vi "Main.vi"() -> ()   [LabVIEW 2015, in "ISA010_module.lvlib"]
doc: "This template is based from the Queued Message Handler design pattern and the Queued Message Handler Project Template that ships with LabVIEW 2014.\n\nThe main difference is that the Queue is private to this module and communication between modules is done via Broadcast and Requests events.\n\nRequests events are wrapped via public API methods and are handled in the Event handler loop in this VI.\nAny module can register for Broadcast events sent by this module.\n\nThe Event Handling Loop generates messages based on user interface actions.\n\nThe Message Handling Loop processes messages generated by the Event Handling Loop, or by other messages. The messages are string values, so new messages can be added easily to the Message Cases case structure in the Message Handling Loop. Each message cluster can also provide an optional value for Message Data, which is a variant that can be converted to whatever message-specific data is required.\n_____\nBased on Delacor QMH Project Template 3.1.0.34."
uses:
  ISA010_module.lvlib
  <vilib>/Delacor/Delacor QMH/Libraries/Cloneable Module Admin_class/Delacor_lib_QMH_Cloneable Module Admin.lvclass
  Module Data--cluster.ctl
  ISA010/ISA010.lvclass
  libraries/ModBUS.lvlibp/ASCII/ASCII.lvclass
  <vilib>/Delacor/Delacor QMH/Libraries/Cloneable Module Admin_class/Delacor_lib_QMH_Cloneable Module Admin.lvclass/Delacor_lib_QMH_Cloneable Module Admin.ctl
  Stop Argument--cluster.ctl
  <vilib>/Delacor/Delacor QMH/Libraries/Module Admin_class/Delacor_lib_QMH_Module Admin.lvclass/Delacor_lib_QMH_Module Admin.ctl
  getISA010State Argument--cluster.ctl
  setPWM Argument--cluster.ctl
  SetServiceMode Argument--cluster.ctl
  setDKG Argument--cluster.ctl
  setKASAWAR Argument--cluster.ctl
  Config Argument--cluster.ctl
  <vilib>/Utility/miscctls.llb/LVPointTypeDef.ctl
  <vilib>/Delacor/Delacor QMH/Libraries/Cloneable Module Admin_class/Delacor_lib_QMH_Get Module ID.vi
  <vilib>/Delacor/Delacor QMH/Libraries/Module Admin_class/Delacor_lib_QMH_Get External Launch.vi
  <vilib>/Delacor/Delacor QMH/Libraries/Message Queue_class/Delacor_lib_QMH_Enqueue Message (Single).vi
  <vilib>/Utility/error.llb/Error Cluster From Error Code.vi
  <vilib>/ErrorRing/Error Ring.xnode
  <vilib>/Delacor/Delacor QMH/Libraries/Message Queue_class/Delacor_lib_QMH_Message Queue.lvclass
  Clone Registration/Clone Registration.lvlib
  libraries/Serializer.lvlibp
  libraries/MQTT.lvlibp
panel:
  in  "Simulate MHL Error":bool
  in  "Simulate EHL Error":bool
  out "error out":errorcluster
  in  "Module Admin":refnum<class "Delacor_lib_QMH_Cloneable Module Admin.lvclass">
  out "Status":string
  # "Other QMH Modules communicate with this Module via its Public API (wrappers for its Request Events).\n\nThis Module communicates with other Modules via its Broadcast Events.\nAny module that wants to get these messages, just registers for this module's Broadcast events."
  # "This template is for the Delacor Modified Queued Message Handler design pattern.\n\nSee the block diagram for more information on how to use this template."
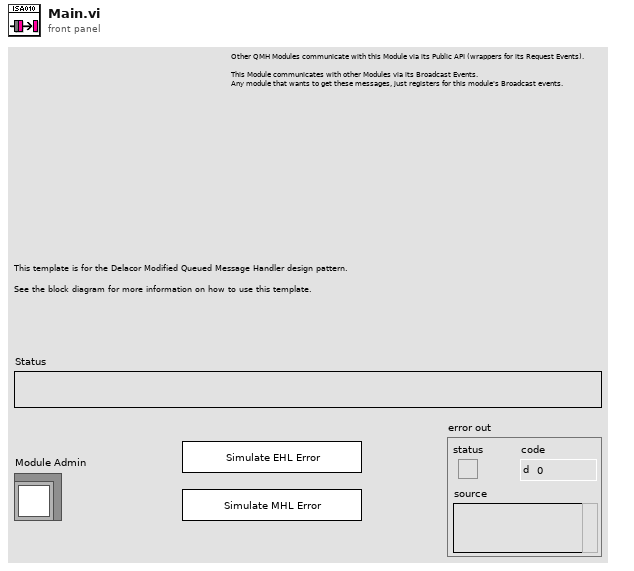
[diagram p1: front panel]
types:
  T1 = typedef "ISA010_module.lvlib/Request Events--cluster.ctl" = cluster{"Stop Module":refnum<user-event>, "Show Panel":refnum<user-event>, "Hide Panel":refnum<user-event>, "Show Diagram":refnum<user-event>, "Get Module Execution Status":refnum<user-event>, "getISA010State":refnum<user-event>, "setPWM":refnum<user-event>, "SetServiceMode":refnum<user-event>, "setDKG":refnum<user-event>, "setKASAWAR":refnum<user-event>, "Config":refnum<user-event>}
  T2 = typedef "Serializer.lvlibp/Broadcast Events--cluster.ctl" = cluster{"Module Did Init":refnum<user-event>, "Status Updated":refnum<user-event>, "Error Reported":refnum<user-event>, "Module Did Stop":refnum<user-event>, "Update Module Execution Status":refnum<user-event>, "Received":refnum<user-event>}
  T3 = typedef "MQTT.lvlibp/Broadcast Events--cluster.ctl" = cluster{"Module Did Init":refnum<user-event>, "Status Updated":refnum<user-event>, "Error Reported":refnum<user-event>, "Module Did Stop":refnum<user-event>, "Update Module Execution Status":refnum<user-event>, "Message":refnum<user-event>}
  T4 = typedef "ISA010_module.lvlib/Module Data--cluster.ctl" = cluster{"Status":string, "Serial Module ID":i32, "ISA010":refnum<class "ISA010.lvclass">, "ISACommands":string[], "ModBUS":refnum<class "ASCII.lvclass">, "outputs":u16, "outputCommand":string}
  T5 = typedef "ISA010_module.lvlib/Stop Argument--cluster.ctl" = cluster{"Origin":string, "Module ID":i32, "Exit via Stop Module Req?":bool, "Wait for Module to stop?":bool}
  T6 = typedef "ISA010_module.lvlib/getISA010State Argument--cluster.ctl" = cluster{"Module ID":i32, "Boolean":bool, "state":string}
  T7 = typedef "ISA010_module.lvlib/setPWM Argument--cluster.ctl" = cluster{"Module ID":i32, "PWM":u8}
  T8 = typedef "ISA010_module.lvlib/SetServiceMode Argument--cluster.ctl" = cluster{"Module ID":i32, "SET":bool}
  T9 = typedef "ISA010_module.lvlib/setDKG Argument--cluster.ctl" = cluster{"Module ID":i32, "DKG":bool}
  T10 = typedef "ISA010_module.lvlib/setKASAWAR Argument--cluster.ctl" = cluster{"Module ID":i32, "KASAWAR":bool}
  T11 = typedef "ISA010_module.lvlib/Config Argument--cluster.ctl" = cluster{"Module ID":i32, "ConfigJson":string}
  T12 = typedef "LVPointTypeDef.ctl" = cluster{"Horizontal":i16, "Vertical":i16}
  T13 = enum32{"Invalid", "Standard", "Closed", "Hidden", "Minimized", "Maximized"}
  T14 = enum32{"invalid lock state", "Not Locked", "Locked (No Password)", "Password-protected"}
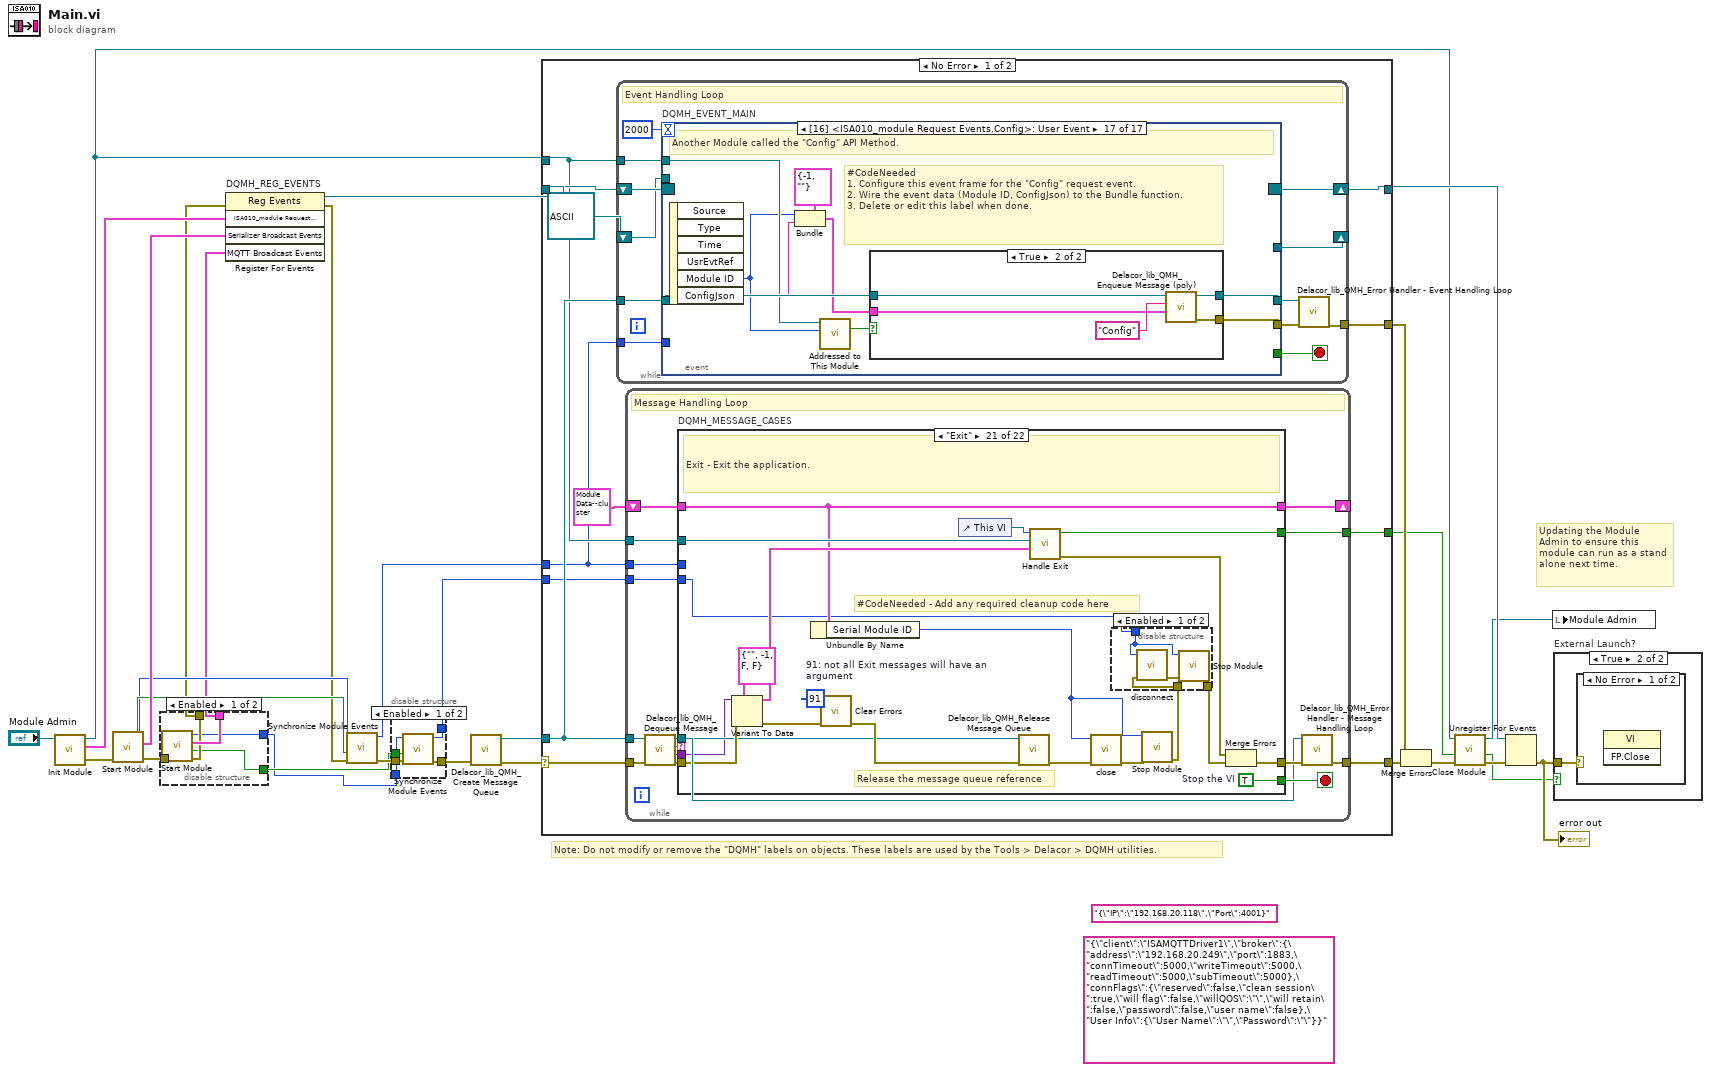
[diagram p0: block diagram]
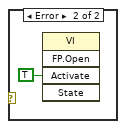
[diagram p5: hidden frame]
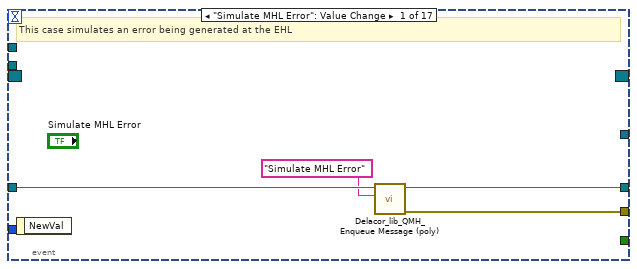
[diagram p6: hidden frame]
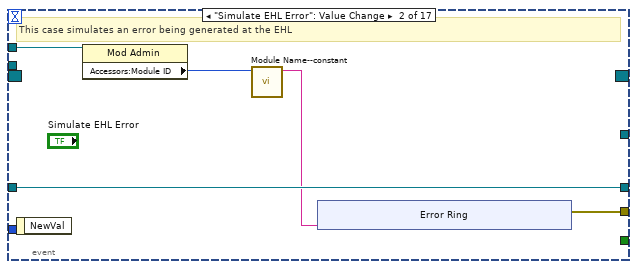
[diagram p7: hidden frame]
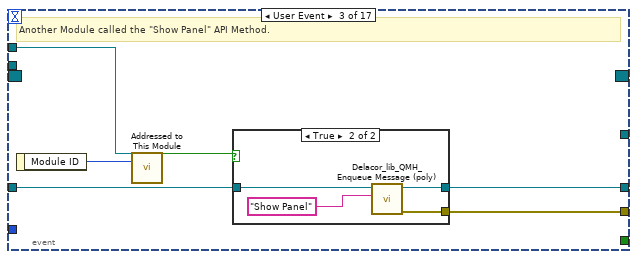
[diagram p8: hidden frame]
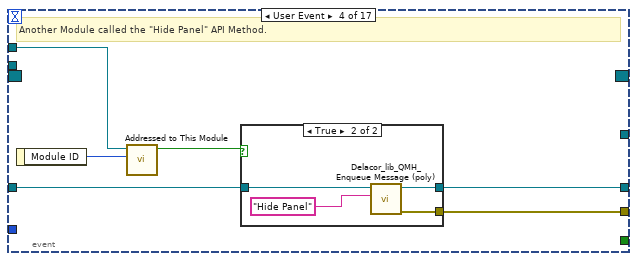
[diagram p10: hidden frame]
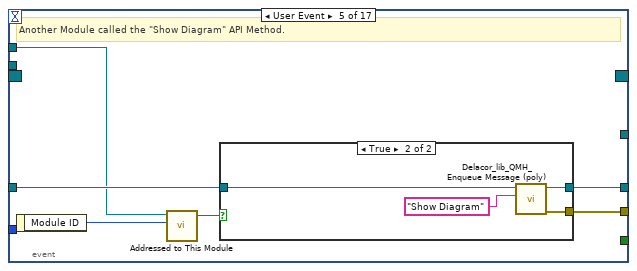
[diagram p12: hidden frame]
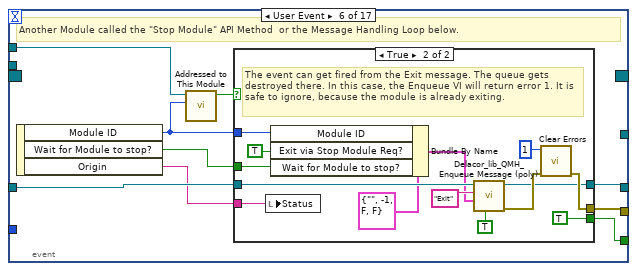
[diagram p14: hidden frame]
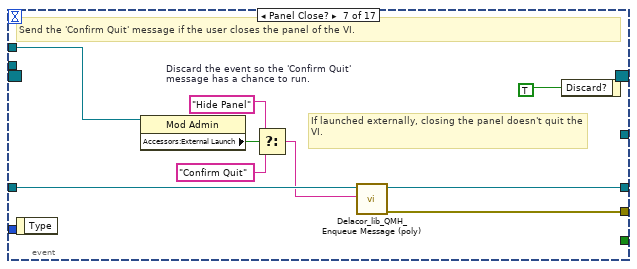
[diagram p16: hidden frame]
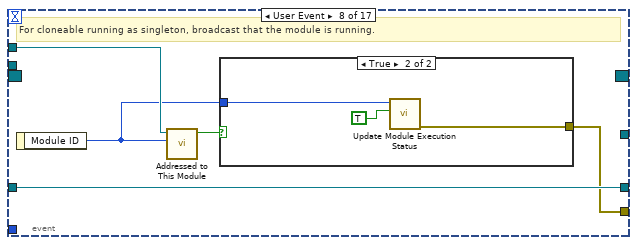
[diagram p17: hidden frame]
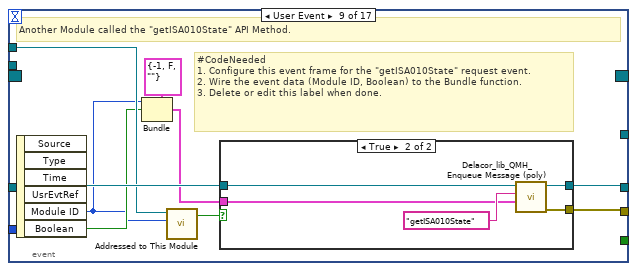
[diagram p19: hidden frame]
diagram:
  (unwired) "{\"IP\":\"192.168.20.118\",\"Port\":4001}" ("config")
  (unwired) "{\"client\":\"ISAMQTTDriver1\",\"broker\":{\"address\":\"192.168.20.249\",\"port\":1883,\"connTimeout\":5000,\"writeTimeout\":5000,\"readTimeout\":5000,\"subTimeout\":5000},\"connFlags\":{\"reserved\":false,\"clean session\":true,\"will flag\":false,\"willQOS\":\"\",\"will retain\":false,\"password\":false,\"user name\":false},\"User Info\":{\"User Name\":\"\",\"Password\":\"\"}}" ("JSON config")
  # "Note: Do not modify or remove the \"DQMH\" labels on objects. These labels are used by the Tools > Delacor > DQMH utilities."
  # "Updating the Module Admin to ensure this module can run as a stand alone next time."
  n1 = call "Init Module.vi"("Cloneable Module Admin in"="Module Admin") -> ("error out"=w16:errorcluster, "ISA010_module Request Events"=w24:T1, "Cloneable Module Admin out"=w21:refnum<class "Delacor_lib_QMH_Cloneable Module Admin.lvclass">)  [unwired: 8 in]
  n2 = call "Start Module.vi"("error in (no error)"=w16) -> ("error out"=w10:errorcluster, "Wait for Event Sync?"=w14:bool, "Serializer Broadcast Events"=w15:T2, "Module ID"=w13:i32)  [unwired: 7 in]
  n3 = disable-structure shown="Enabled" {
    disable-tunnel: w10 -> [w34 w35]
    disable-tunnel: [w33 _] -> w9
    disable-tunnel: [w32 w35] -> w8
    disable-tunnel: [w31 _] -> w5
    disable-tunnel: [w30 _] -> w4
    frame Enabled {
      n4 = call "Start Module.vi"("error in (no error)"=w34) -> ("error out"=w32:errorcluster, "Wait for Event Sync?"=w31:bool, "MQTT Broadcast Events"=w33:T3, "Module ID"=w30:i32)  [unwired: 7 in]
    }
    frame Disabled {
    }
  }
  n5 = register-events "DQMH_REG_EVENTS"(error in=w8, w24, w15, w9) -> (reference out=w25:refnum<event-registration>, error out=w12:errorcluster)  [unwired: 1 in]
  n6 = call "Synchronize Module Events.vi"("error in (no error)"=w12, "Wait for Event Sync?"=w14, "Module ID"=w13) -> ("error out"=w7:errorcluster, "Module ID (dup)"=w11:i32)  [unwired: 7 in]
  n7 = disable-structure shown="Enabled" {
    disable-tunnel: w7 -> [w40 _]
    disable-tunnel: [w39 _] -> w6
    disable-tunnel: w5 -> [w38 _]
    disable-tunnel: w4 -> [w37 _]
    disable-tunnel: [w36 _] -> w3
    frame Enabled {
      n8 = call "Synchronize Module Events.vi"("error in (no error)"=w40, "Wait for Event Sync?"=w38, "Module ID"=w37) -> ("error out"=w39:errorcluster, "Module ID (dup)"=w36:i32)  [unwired: 7 in]
    }
    frame Disabled {
    }
  }
  n9 = call <vilib>:"Delacor_lib_QMH_Create Message Queue.vi"("error in (no error)"=w6) -> ("error out"=w1:errorcluster, "Message Queue out"=w2:refnum<class "Delacor_lib_QMH_Message Queue.lvclass">)  [unwired: 9 in]
  n10 = case shown="No Error" w1 {
    selector: w1 -> [w46 w709]
    tunnel: [w52 w709] -> w27
    tunnel: [w51 w710] -> w26
    tunnel: w25 -> [w49 w710]
    tunnel: w2 -> [w48 _]
    tunnel: [w47 _] -> w28
    tunnel: w21 -> [w45 w705]
    tunnel: [w44 _] -> w19
    tunnel: w11 -> [w43 _]
    tunnel: w3 -> [w41 _]
    frame No Error {
      n11 = while {
        tunnel: w48 -> [w64]
        shift-right: [w62] -> w51
        shift-left: w49 -> [w63]
        tunnel: [w58] -> w47
        tunnel: w45 -> [w57]
        shift-right: [w55] -> _
        shift-left: refnum<class "ASCII.lvclass"> refnum ("ModBUS.lvlibp:ASCII.lvclass") -> [w56]
        tunnel: w43 -> [w54]
        stop <- w60 stop-if-true
        # "Event Handling Loop"
        n12 = event "DQMH_EVENT_MAIN" shown="[16] <ISA010_module Request Events.Config>: User Event" {
          selector: w63 -> [_ _ _ _ _ _ _ _ _ _ _ _ _ _ _ _ _]
          dyn-events: [_ _ _ _ _ _ _ _ _ _ _ _ _ _ _ _ _] -> w62
          timeout: 2000 -> [_ _ _ _ _ _ _ _ _ _ _ _ _ _ _ _ _]
          tunnel: [_ _ _ _ _ w117 _ _ _ _ _ _ _ _ _ _ _] -> w60
          tunnel: w64 -> [w68 w73 w86 w97 w108 w120 w145 w149 w163 w174 w205 w220 w228 w238 w253 w261 w308]
          tunnel: [w66 w72 w84 w95 w104 w122 w144 w148 w157 _ w199 w214 _ w232 w247 _ w302] -> w61
          tunnel: [w67 w73 w85 w96 w107 w121 w143 w149 w162 w173 w204 w219 w227 w237 w252 w262 w307] -> w59
          tunnel: w57 -> [_ w71 w81 w92 w105 w119 w139 w150 w160 _ w202 w217 _ w235 w250 _ w305]
          tunnel: w56 -> [_ _ _ _ _ _ _ _ _ w176 _ _ _ _ _ _ _]
          tunnel: [_ _ _ _ _ _ _ _ _ w175 _ _ _ _ _ _ _] -> w55
          tunnel: w54 -> [_ _ _ _ _ _ _ _ _ w170 _ _ _ _ _ _ _]
          event "Simulate MHL Error": Value Change {
            # "This case simulates an error being generated at the EHL"
            n13 = event-data() -> ()  [unwired: 1 in, 1 out]
            n14 = call-poly <vilib>:"Delacor_lib_QMH_Enqueue Message (poly).vi"("Message"="Simulate MHL Error", "Message Queue in"=w68) -> ("error out"=w66:errorcluster, "Message Queue out"=w67:refnum<class "Delacor_lib_QMH_Message Queue.lvclass">)  [unwired: 8 in]
          }
          event "Simulate EHL Error": Value Change {
            # "This case simulates an error being generated at the EHL"
            n15 = event-data() -> ()  [unwired: 1 in, 1 out]
            n16 = property class="Mod Admin"(reference=w71) -> ("Accessors:Module ID"=w70:i32)  [unwired: 1 in, 2 out]
            n17 = call "Module Name--constant.vi"("Module ID"=w70) -> ("Module Name"=w69:string)  [unwired: 10 in]
            n18 = xnode "Error Ring"("parameter 0"=w69) -> ("error out"=w72:errorcluster)
          }
          event User Event {
            # "Another Module called the \"Show Panel\" API Method."
            n19 = event-data() -> ("Module ID"=w83:i32)  [unwired: 1 in]
            n20 = call "Addressed to This Module.vi"("Module ID from Argument"=w83, "Module Admin"=w81) -> ("Addressed to this instance?"=w82:bool)  [unwired: 8 in, 1 out]
            n21 = case shown="True" w82 {
              tunnel: w86 -> [w87 w91]
              tunnel: [w87 w90] -> w85
              tunnel: [_ w89] -> w84
              frame False {
              }
              frame True {
                n22 = call-poly <vilib>:"Delacor_lib_QMH_Enqueue Message (poly).vi"("Message"="Show Panel", "Message Queue in"=w91) -> ("error out"=w89:errorcluster, "Message Queue out"=w90:refnum<class "Delacor_lib_QMH_Message Queue.lvclass">)  [unwired: 8 in]
              }
            }
          }
          event User Event {
            # "Another Module called the \"Hide Panel\" API Method."
            n23 = event-data() -> ("Module ID"=w94:i32)  [unwired: 1 in]
            n24 = call "Addressed to This Module.vi"("Module ID from Argument"=w94, "Module Admin"=w92) -> ("Addressed to this instance?"=w93:bool)  [unwired: 8 in, 1 out]
            n25 = case shown="True" w93 {
              tunnel: w97 -> [w98 w102]
              tunnel: [w98 w101] -> w96
              tunnel: [_ w100] -> w95
              frame False {
              }
              frame True {
                n26 = call-poly <vilib>:"Delacor_lib_QMH_Enqueue Message (poly).vi"("Message"="Hide Panel", "Message Queue in"=w102) -> ("error out"=w100:errorcluster, "Message Queue out"=w101:refnum<class "Delacor_lib_QMH_Message Queue.lvclass">)  [unwired: 8 in]
              }
            }
          }
          event User Event {
            # "Another Module called the \"Show Diagram\" API Method."
            n27 = event-data() -> ("Module ID"=w103:i32)  [unwired: 1 in]
            n28 = call "Addressed to This Module.vi"("Module ID from Argument"=w103, "Module Admin"=w105) -> ("Addressed to this instance?"=w106:bool)  [unwired: 8 in, 1 out]
            n29 = case shown="True" w106 {
              tunnel: w108 -> [w109 w113]
              tunnel: [w109 w112] -> w107
              tunnel: [_ w110] -> w104
              frame False {
              }
              frame True {
                n30 = call-poly <vilib>:"Delacor_lib_QMH_Enqueue Message (poly).vi"("Message"="Show Diagram", "Message Queue in"=w113) -> ("error out"=w110:errorcluster, "Message Queue out"=w112:refnum<class "Delacor_lib_QMH_Message Queue.lvclass">)  [unwired: 8 in]
              }
            }
          }
          event User Event {
            # "Another Module called the \"Stop Module\" API Method  or the Message Handling Loop below."
            n31 = event-data() -> ("Module ID"=w115:i32, "Wait for Module to stop?"=w116:bool, "Origin"=w114:string)  [unwired: 1 in]
            n32 = call "Addressed to This Module.vi"("Module ID from Argument"=w115, "Module Admin"=w119) -> ("Addressed to this instance?"=w118:bool)  [unwired: 8 in, 1 out]
            n33 = case shown="True" w118 {
              tunnel: [_ w133] -> w122
              tunnel: [w123 w132] -> w121
              tunnel: w120 -> [w123 w131]
              tunnel: [_ TRUE] -> w117
              tunnel: w116 -> [_ w126]
              tunnel: w115 -> [_ w128]
              tunnel: w114 -> [_ w124]
              frame False {
              }
              frame True {
                # "The event can get fired from the Exit message. The queue gets destroyed there. In this case, the Enqueue VI will return error 1. It is safe to ignore, because the module is already exiting."
                n34 = local write "Status"(w124) -> ()
                n35 = Bundle By Name(cluster=T5 {"Origin"="", "Module ID"=-1, "Exit via Stop Module Req?"=FALSE, "Wait for Module to stop?"=FALSE} ("Stop Argument"), "Module ID"=w128, "Exit via Stop Module Req?"=TRUE, "Wait for Module to stop?"=w126) -> (w125:T5)
                n36 = call-poly <vilib>:"Delacor_lib_QMH_Enqueue Message (poly).vi"("Priority Message? (F)"=TRUE, "Message Data"=w125, "Message"="Exit", "Message Queue in"=w131) -> ("error out"=w136:errorcluster, "Message Queue out"=w132:refnum<class "Delacor_lib_QMH_Message Queue.lvclass">)  [unwired: 6 in]
                n37 = call <vilib>:"Clear Errors.vi"("error in (no error)"=w136, "specific error code to clear (0: all)"=1) -> ("error out"=w133:errorcluster)  [unwired: 4 in, 1 out]
              }
            }
          }
          event Panel Close? {
            w146 = TRUE  # Discard the event so the 'Confirm Quit' message has a chance to run.
            # "If launched externally, closing the panel doesn't quit the VI."
            # "Send the 'Confirm Quit' message if the user closes the panel of the VI."
            n38 = event-data() -> ()  [unwired: 1 in, 1 out]
            n39 = property class="Mod Admin"(reference=w139) -> ("Accessors:External Launch"=w138:bool)  [unwired: 1 in, 2 out]
            n40 = Select(t="Hide Panel" ("Message"), s=w138, f="Confirm Quit" ("Message")) -> (s? t:f=w140:string)
            n41 = call-poly <vilib>:"Delacor_lib_QMH_Enqueue Message (poly).vi"("Message"=w140, "Message Queue in"=w145) -> ("error out"=w144:errorcluster, "Message Queue out"=w143:refnum<class "Delacor_lib_QMH_Message Queue.lvclass">)  [unwired: 8 in]
            n42 = event-data("Discard?"=w146) -> ()  [unwired: 1 in, 1 out]
          }
          event User Event {
            # "For cloneable running as singleton, broadcast that the module is running."
            n43 = event-data() -> ("Module ID"=w147:i32)  [unwired: 1 in]
            n44 = call "Addressed to This Module.vi"("Module ID from Argument"=w147, "Module Admin"=w150) -> ("Addressed to this instance?"=w151:bool)  [unwired: 8 in, 1 out]
            n45 = case shown="True" w151 {
              tunnel: [_ w154] -> w148
              tunnel: w147 -> [_ w153]
              frame False {
              }
              frame True {
                n46 = call "Update Module Execution Status.vi"("Running?"=TRUE, "Module ID"=w153) -> ("error out"=w154:errorcluster)  [unwired: 9 in]
              }
            }
          }
          event User Event {
            # "#CodeNeeded\n1. Configure this event frame for the \"getISA010State\" request event.\n2. Wire the event data (Module ID, Boolean) to the Bundle function.\n3. Delete or edit this label when done."
            # "Another Module called the \"getISA010State\" API Method."
            n47 = event-data() -> ("Module ID"=w155:i32, "Boolean"=w156:bool)  [unwired: 1 in, 4 out]
            n48 = Bundle(cluster=T6 {"Module ID"=-1, "Boolean"=FALSE, "state"=""} ("getISA010State Argument"), "Module ID"=w155, "Boolean"=w156) -> (w158:T6)  [unwired: 1 in]
            n49 = call "Addressed to This Module.vi"("Module ID from Argument"=w155, "Module Admin"=w160) -> ("Addressed to this instance?"=w161:bool)  [unwired: 8 in, 1 out]
            n50 = case shown="True" w161 {
              tunnel: w163 -> [w164 w169]
              tunnel: [w164 w168] -> w162
              tunnel: w158 -> [_ w166]
              tunnel: [_ w165] -> w157
              frame False {
              }
              frame True {
                n51 = call-poly <vilib>:"Delacor_lib_QMH_Enqueue Message (poly).vi"("Message Data"=w166, "Message"="getISA010State", "Message Queue in"=w169) -> ("error out"=w165:errorcluster, "Message Queue out"=w168:refnum<class "Delacor_lib_QMH_Message Queue.lvclass">)  [unwired: 7 in]
              }
            }
          }
          event User Event {
            n52 = event-data() -> ("Module ID"=w171:i32, "Bytes"=w177:u8[])  [unwired: 1 in, 4 out]
            n53 = Equal?(x=w171, y=w170) -> (x = y?=w172:bool)
            n54 = case shown="True" w172 {
              tunnel: w177 -> [_ w184]
              tunnel: w176 -> [w179 w183]
              tunnel: [w179 w182] -> w175
              tunnel: w174 -> [w178 w181]
              tunnel: [w178 w180] -> w173
              frame False {
              }
              frame True {
                n55 = for {
                  tunnel: w184 -> [w191] mode=indexing
                  shift-right: [w189] -> w182
                  shift-left: w183 -> [w190]
                  shift-right: [w185] -> w180
                  shift-left: w181 -> [w186]
                  n56 = call-dynamic "collectFrame.vi"("byte"=w191, "ASCII in"=w190) -> ("Data"=w187:i16[], "Finished"=w188:bool, "ASCII out"=w189:refnum<class "ASCII.lvclass">)  [unwired: 5 in, 2 out]
                  n57 = case shown="True" w188 {
                    tunnel: w187 -> [_ w193]
                    tunnel: w186 -> [w192 w196]
                    tunnel: [w192 w195] -> w185
                    frame False {
                    }
                    frame True {
                      n58 = call-poly <vilib>:"Delacor_lib_QMH_Enqueue Message (poly).vi"("Message Data"=w193, "Message"="ModbusReply", "Message Queue in"=w196) -> ("Message Queue out"=w195:refnum<class "Delacor_lib_QMH_Message Queue.lvclass">)  [unwired: 7 in, 1 out]
                    }
                  }
                }
              }
            }
          }
          event User Event {
            # "#CodeNeeded\n1. Configure this event frame for the \"setPWM\" request event.\n2. Wire the event data (Module ID, PWM) to the Bundle function.\n3. Delete or edit this label when done."
            # "Another Module called the \"setPWM\" API Method."
            n59 = event-data() -> ("Module ID"=w197:i32, "PWM"=w198:u8)  [unwired: 1 in, 4 out]
            n60 = Bundle(cluster=T7 {"Module ID"=-1, "PWM"=0} ("setPWM Argument"), "Module ID"=w197, "PWM"=w198) -> (w200:T7)
            n61 = call "Addressed to This Module.vi"("Module ID from Argument"=w197, "Module Admin"=w202) -> ("Addressed to this instance?"=w203:bool)  [unwired: 8 in, 1 out]
            n62 = case shown="True" w203 {
              tunnel: w205 -> [w206 w211]
              tunnel: [w206 w210] -> w204
              tunnel: w200 -> [_ w208]
              tunnel: [_ w207] -> w199
              frame False {
              }
              frame True {
                n63 = call-poly <vilib>:"Delacor_lib_QMH_Enqueue Message (poly).vi"("Message Data"=w208, "Message"="setPWM", "Message Queue in"=w211) -> ("error out"=w207:errorcluster, "Message Queue out"=w210:refnum<class "Delacor_lib_QMH_Message Queue.lvclass">)  [unwired: 7 in]
              }
            }
          }
          event User Event {
            # "#CodeNeeded\n1. Configure this event frame for the \"SetServiceMode\" request event.\n2. Wire the event data (Module ID, SET) to the Bundle function.\n3. Delete or edit this label when done."
            # "Another Module called the \"SetServiceMode\" API Method."
            n64 = event-data() -> ("Module ID"=w213:i32, "SET"=w212:bool)  [unwired: 1 in, 4 out]
            n65 = Bundle(cluster=T8 {"Module ID"=-1, "SET"=FALSE} ("SetServiceMode Argument"), "Module ID"=w213, "SET"=w212) -> (w215:T8)
            n66 = call "Addressed to This Module.vi"("Module ID from Argument"=w213, "Module Admin"=w217) -> ("Addressed to this instance?"=w218:bool)  [unwired: 8 in, 1 out]
            n67 = case shown="True" w218 {
              tunnel: w220 -> [w221 w226]
              tunnel: [w221 w225] -> w219
              tunnel: w215 -> [_ w223]
              tunnel: [_ w222] -> w214
              frame False {
              }
              frame True {
                n68 = call-poly <vilib>:"Delacor_lib_QMH_Enqueue Message (poly).vi"("Message Data"=w223, "Message"="SetServiceMode", "Message Queue in"=w226) -> ("error out"=w222:errorcluster, "Message Queue out"=w225:refnum<class "Delacor_lib_QMH_Message Queue.lvclass">)  [unwired: 7 in]
              }
            }
          }
          event Timeout {
            n69 = event-data() -> ()  [unwired: 1 in, 3 out]
            n70 = call-poly <vilib>:"Delacor_lib_QMH_Enqueue Message (poly).vi"("Message"="getISA010State", "Message Queue in"=w228) -> ("Message Queue out"=w227:refnum<class "Delacor_lib_QMH_Message Queue.lvclass">)  [unwired: 8 in, 1 out]
          }
          event User Event {
            # "#CodeNeeded\n1. Configure this event frame for the \"setDKG\" request event.\n2. Wire the event data (Module ID, DKG) to the Bundle function.\n3. Delete or edit this label when done."
            # "Another Module called the \"setDKG\" API Method."
            n71 = event-data() -> ("Module ID"=w230:i32, "DKG"=w231:bool)  [unwired: 1 in, 4 out]
            n72 = Bundle(cluster=T9 {"Module ID"=-1, "DKG"=FALSE} ("setDKG Argument"), "Module ID"=w230, "DKG"=w231) -> (w233:T9)
            n73 = call "Addressed to This Module.vi"("Module ID from Argument"=w230, "Module Admin"=w235) -> ("Addressed to this instance?"=w236:bool)  [unwired: 8 in, 1 out]
            n74 = case shown="True" w236 {
              tunnel: w238 -> [w239 w244]
              tunnel: [w239 w243] -> w237
              tunnel: w233 -> [_ w241]
              tunnel: [_ w240] -> w232
              frame False {
              }
              frame True {
                n75 = call-poly <vilib>:"Delacor_lib_QMH_Enqueue Message (poly).vi"("Message Data"=w241, "Message"="setDKG", "Message Queue in"=w244) -> ("error out"=w240:errorcluster, "Message Queue out"=w243:refnum<class "Delacor_lib_QMH_Message Queue.lvclass">)  [unwired: 7 in]
              }
            }
          }
          event User Event {
            # "#CodeNeeded\n1. Configure this event frame for the \"setKASAWAR\" request event.\n2. Wire the event data (Module ID, KASAWAR) to the Bundle function.\n3. Delete or edit this label when done."
            # "Another Module called the \"setKASAWAR\" API Method."
            n76 = event-data() -> ("Module ID"=w245:i32, "KASAWAR"=w246:bool)  [unwired: 1 in, 4 out]
            n77 = Bundle(cluster=T10 {"Module ID"=-1, "KASAWAR"=FALSE} ("setKASAWAR Argument"), "Module ID"=w245, "KASAWAR"=w246) -> (w248:T10)
            n78 = call "Addressed to This Module.vi"("Module ID from Argument"=w245, "Module Admin"=w250) -> ("Addressed to this instance?"=w251:bool)  [unwired: 8 in, 1 out]
            n79 = case shown="True" w251 {
              tunnel: w253 -> [w254 w259]
              tunnel: [w254 w258] -> w252
              tunnel: w248 -> [_ w256]
              tunnel: [_ w255] -> w247
              frame False {
              }
              frame True {
                n80 = call-poly <vilib>:"Delacor_lib_QMH_Enqueue Message (poly).vi"("Message Data"=w256, "Message"="setKASAWAR", "Message Queue in"=w259) -> ("error out"=w255:errorcluster, "Message Queue out"=w258:refnum<class "Delacor_lib_QMH_Message Queue.lvclass">)  [unwired: 7 in]
              }
            }
          }
          event User Event {
            n81 = event-data() -> ("Topic"=w263:string, "Message"=w260:string)  [unwired: 1 in, 5 out]
            n82 = case shown="\"ISA010\\\\KASAWAR\"" w263 {
              tunnel: [w264 w266 w274 w294] -> w262
              tunnel: w261 -> [w264 w267 w275 w295]
              tunnel: w260 -> [_ w271 w279 w297]
              frame "False", Default {
              }
              frame "ISA010\\DKG" {
                n83 = case shown="\"0\", \"False\", Default" w271 {
                  tunnel: [FALSE ("DKG") TRUE ("DKG")] -> w269
                  frame "0", "False", Default {
                  }
                  frame "1", "True" {
                  }
                }
                n84 = Bundle(cluster=T9 {"Module ID"=-1, "DKG"=FALSE} ("setDKG Argument"), "DKG"=w269) -> (w265:T9)  [unwired: 1 in]
                n85 = call-poly <vilib>:"Delacor_lib_QMH_Enqueue Message (poly).vi"("Message Data"=w265, "Message"="setDKG", "Message Queue in"=w267) -> ("Message Queue out"=w266:refnum<class "Delacor_lib_QMH_Message Queue.lvclass">)  [unwired: 7 in, 1 out]
              }
              frame "ISA010\\PWM" {
                n86 = Scan From String(format string="%d", input string=w279) -> (error out=w277:errorcluster, output 1=w276:i32)  [unwired: 3 in, 2 out]
                n87 = case shown="No Error" w277 {
                  tunnel: w276 -> [w289 _]
                  tunnel: w275 -> [w281 w290]
                  tunnel: [w280 w290] -> w274
                  frame No Error {
                    n88 = In Range and Coerce(upper limit=100, x=w289, lower limit=0) -> (coerced(x)=w284:i32)  [unwired: 1 out]
                    n89 = Bundle(cluster=T7 {"Module ID"=-1, "PWM"=0} ("setPWM Argument"), "Module ID"=0, "PWM"=w284) -> (w283:T7)
                    n90 = call-poly <vilib>:"Delacor_lib_QMH_Enqueue Message (poly).vi"("Message Data"=w283, "Message"="setPWM", "Message Queue in"=w281) -> ("Message Queue out"=w280:refnum<class "Delacor_lib_QMH_Message Queue.lvclass">)  [unwired: 7 in, 1 out]
                  }
                  frame Error {
                  }
                }
              }
              frame "ISA010\\KASAWAR" {
                n91 = case shown="\"0\", \"False\", Default" w297 {
                  tunnel: [FALSE ("DKG") TRUE ("DKG")] -> w296
                  frame "0", "False", Default {
                  }
                  frame "1", "True" {
                  }
                }
                n92 = Bundle(cluster=T10 {"Module ID"=-1, "KASAWAR"=FALSE} ("setKASAWAR Argument"), "KASAWAR"=w296) -> (w293:T10)  [unwired: 1 in]
                n93 = call-poly <vilib>:"Delacor_lib_QMH_Enqueue Message (poly).vi"("Message Data"=w293, "Message"="setKASAWAR", "Message Queue in"=w295) -> ("Message Queue out"=w294:refnum<class "Delacor_lib_QMH_Message Queue.lvclass">)  [unwired: 7 in, 1 out]
              }
            }
          }
          event User Event {
            # "#CodeNeeded\n1. Configure this event frame for the \"Config\" request event.\n2. Wire the event data (Module ID, ConfigJson) to the Bundle function.\n3. Delete or edit this label when done."
            # "Another Module called the \"Config\" API Method."
            n94 = event-data() -> ("Module ID"=w301:i32, "ConfigJson"=w300:string)  [unwired: 1 in, 4 out]
            n95 = Bundle(cluster=T11 {"Module ID"=-1, "ConfigJson"=""} ("Config Argument"), "Module ID"=w301, "ConfigJson"=w300) -> (w303:T11)
            n96 = call "Addressed to This Module.vi"("Module ID from Argument"=w301, "Module Admin"=w305) -> ("Addressed to this instance?"=w306:bool)  [unwired: 8 in, 1 out]
            n97 = case shown="True" w306 {
              tunnel: w308 -> [w309 w314]
              tunnel: [w309 w313] -> w307
              tunnel: w303 -> [_ w311]
              tunnel: [_ w310] -> w302
              frame False {
              }
              frame True {
                n98 = call-poly <vilib>:"Delacor_lib_QMH_Enqueue Message (poly).vi"("Message Data"=w311, "Message"="Config", "Message Queue in"=w314) -> ("error out"=w310:errorcluster, "Message Queue out"=w313:refnum<class "Delacor_lib_QMH_Message Queue.lvclass">)  [unwired: 7 in]
              }
            }
          }
        }
        n99 = call-dynamic "Delacor_lib_QMH_Error Handler - Event Handling Loop.vi"("error in (no error)"=w61, "Message Queue in"=w59) -> ("dup error in"=w58:errorcluster)  [unwired: 8 in, 1 out]
      }
      n100 = while {
        tunnel: w48 -> [w321]
        shift-right: [w327] -> _
        shift-left: T4 {"Status"="", "Serial Module ID"=0, "ISA010"=refnum, "ISACommands"=[], "ModBUS"=refnum, "outputs"=0, "outputCommand"=""} ("Data Cluster") -> [w328]
        tunnel: w46 -> [w325]
        tunnel: [w319] -> w52
        tunnel: w45 -> [w318]
        tunnel: [w317] -> w44
        tunnel: w43 -> [w316]
        tunnel: w41 -> [w315]
        stop <- w326 stop-if-true
        # "Message Handling Loop"
        n101 = call-dynamic "Delacor_lib_QMH_Dequeue Message.vi"("error in (no error)"=w325, "Message Queue in"=w321) -> ("error out"=w324:errorcluster, "Message Data"=w322:variant, "Message"=w323:string, "Message Queue out"=w320:refnum<class "Delacor_lib_QMH_Message Queue.lvclass">)  [unwired: 6 in]
        n102 = case "DQMH_MESSAGE_CASES" shown="\"Exit\"" w323 {
          selector: w323 -> [_ _ _ _ _ _ _ _ _ _ _ _ _ _ _ _ _ _ _ _ _ w692]
          tunnel: w320 -> [_ _ _ _ _ _ _ _ _ _ _ w525 w543 w562 _ w578 _ w626 _ w659 w681 _]
          tunnel: w324 -> [w345 w361 w369 w375 w378 w399 w419 w438 w461 w482 w523 w538 w553 w574 w577 w586 w624 w635 w648 w658 w683 _]
          tunnel: [w332 w362 w369 w375 w377 w397 w415 w437 w439 w465 w503 w527 w545 w566 w575 w593 w622 w625 w646 w657 w679 w693] -> w329
          tunnel: w328 -> [w344 w363 w368 w374 w379 w398 w405 w432 w453 w478 w516 w537 w552 w570 w576 w590 w623 w634 w647 w662 w668 w694]
          tunnel: [w343 w363 w368 w374 w379 w398 w404 w431 w452 w477 w515 w533 w549 w570 w576 w580 w623 w634 w647 w662 w668 w694] -> w327
          tunnel: [_ _ _ _ _ _ _ _ _ _ _ _ _ _ _ _ _ _ _ _ w680 _] -> w326
          tunnel: w322 -> [_ w360 _ _ _ _ w418 _ w460 _ w522 w536 w551 w573 _ w583 _ w633 _ _ w675 _]
          tunnel: w318 -> [w337 w355 w366 w373 w376 _ _ _ _ _ _ _ _ _ _ w585 _ w630 w643 _ w671 w690]
          tunnel: [_ _ _ _ _ _ _ _ _ _ _ _ _ _ _ _ _ _ _ _ w673 _] -> w317
          tunnel: w316 -> [w334 _ _ _ _ _ _ _ _ _ _ _ _ _ _ _ _ _ _ _ _ _]
          tunnel: w315 -> [_ _ _ _ _ _ _ _ _ _ _ _ _ w565 _ _ _ _ _ _ w664 _]
          frame "Initialize" {
            w342 = "Initial Message" ("Initial Message")
            # "Initialize - Any operation that needs to be done before the module can receive messages. Synchronize Caller Events.vi will inform Start Module.vi that the module has launched and is ready to receive messages. Module Did Init.vi will broadcast that the module initialized."
            n103 = call "Synchronize Caller Events.vi"("error in (no error)"=w345, "Module Admin"=w337) -> ("error out"=w333:errorcluster, "Module Admin out"=w336:refnum<class "Delacor_lib_QMH_Cloneable Module Admin.lvclass">)  [unwired: 8 in]
            n104 = property on="Pane" class="Pane"("Origin"=T12 {"Horizontal"=0, "Vertical"=0}) -> ()  [unwired: 2 in, 2 out]
            n105 = property class="Mod Admin"(reference=w336, error in=w333) -> (error out=w331:errorcluster, "Accessors:Module ID"=w339:i32, "Accessors:External Launch"=w338:bool)  [unwired: 1 out]
            n106 = call "Module Name--constant.vi"("Module ID"=w339) -> ("Module Name"=w349:string)  [unwired: 10 in]
            n107 = property class="VI"(error in=w331, "Front Panel.Title"=w349) -> (reference out=w352:refnum<vi>, error out=w353:errorcluster)  [unwired: 1 in]
            n108 = Select(t=T13."Hidden" ("State"), s=w338, f=T13."Standard" ("State")) -> (s? t:f=w346:T13)
            n109 = local write "Status"(w342) -> ()
            n110 = invoke class="VI" method="FP.Open"(reference=w352, error in=w353, "State"=w346) -> (reference out=w351:refnum<vi>, error out=w350:errorcluster)  [unwired: 2 in, 3 out]
            n111 = call "Module Name--constant.vi"("Module ID"=w339) -> ("Module Name"=w340:string)  [unwired: 10 in]
            n112 = Bundle By Name(cluster=w344, "Status"=w342, "Serial Module ID"=w334) -> (w343:T4)
            n113 = invoke class="VI" method="FP.Center"(reference=w351, error in=w350) -> (error out=w330:errorcluster)  [unwired: 1 in, 2 out]
            n114 = call "Module Did Init.vi"("error in (no error)"=w330, "Initialized?"=TRUE, "Origin"=w340, "Module ID"=w339) -> ("error out"=w332:errorcluster)  [unwired: 7 in]
          }
          frame "Update Display" {
            # "Broadcast updated status to any VI registered to listen to this module's broadcast events."
            # "Convert the message data to a string to display in the Status indicator."
            # "#CodeRecommended - If you wish to decouple the Message Handling Loop from your user interface, consider creating User Events (like the \"Stop\" event in this VI) to message the Event Handling Loop whenever the user interface needs updating."
            # "Update Display - Update user interface here."
            n115 = Variant To Data(error in=w361, type="", Variant=w360) -> (data=w358:string, error out=w357:errorcluster)
            "Status" <- w358
            n116 = property class="Mod Admin"(reference=w355) -> ("Accessors:Module ID"=w354:i32)  [unwired: 1 in, 2 out]
            n117 = call "Status Updated.vi"("error in (no error)"=w357, "Status"=w358, "Module ID"=w354) -> ("error out"=w356:errorcluster)  [unwired: 8 in]
            n118 = Merge Errors(w356) -> (w362:errorcluster)
          }
          frame "Show Panel" {
            # "Show the panel of this VI, and send a status updated message to let listeners know."
            n119 = property class="Mod Admin"(reference=w366) -> ("Accessors:Module ID"=w365:i32)  [unwired: 1 in, 2 out]
            n120 = call "Status Updated.vi"("Status"="Panel shown." ("format string"), "Module ID"=w365) -> ()  [unwired: 9 in, 1 out]
            n121 = invoke class="VI" method="FP.Open"("Activate"=TRUE ("Activate?")) -> ()  [unwired: 4 in, 5 out]
          }
          frame "Hide Panel" {
            # "Hide the panel of this VI, and send a status updated message to let listeners know."
            n122 = property class="Mod Admin"(reference=w373) -> ("Accessors:Module ID"=w372:i32)  [unwired: 1 in, 2 out]
            n123 = call "Status Updated.vi"("Status"="Panel hidden." ("format string"), "Module ID"=w372) -> ()  [unwired: 9 in, 1 out]
            n124 = invoke class="VI" method="FP.Open"("State"=T13."Hidden") -> ()  [unwired: 4 in, 5 out]
          }
          frame "Show Diagram" {
            # "Show Diagram - Show the block diagram of this VI. Used as a debugging tool. There is a button in the module tester that fires the Show Diagram request, which runs this message. Note that the diagram will not be displayed if it is password-protected and the password is not in the cache."
            n125 = disable-structure shown="RUN_TIME_ENGINE==False" {
              disable-tunnel: [w388 w396] -> w377
              disable-tunnel: w378 -> [w387 w396]
              disable-tunnel: w376 -> [w380 _]
              frame condition #0 (active) {
                # "functionality not available in exe"
                n126 = invoke class="VI" method="Lock State.Get"(error in=w387) -> (error out=w386:errorcluster, "Get Lock State"=w385:T14, "pwd in cache"=w382:bool)  [unwired: 3 in, 1 out]
                n127 = Equal?(x=T14."Password-protected", y=w385) -> (x = y?=w383:bool)
                n128 = Compound Arithmetic op=AND(w383, invert w382) -> (w381:bool)
                n129 = case shown="False" w381 {
                  tunnel: [w393 w395] -> w388
                  tunnel: w386 -> [w392 w395]
                  tunnel: w380 -> [w389 _]
                  frame False {
                    n130 = property class="Mod Admin"(reference=w389) -> ("Accessors:Module ID"=w390:i32)  [unwired: 1 in, 2 out]
                    n131 = property class="VI"(error in=w392, "BDWin.Open"=TRUE ("Block Diagram Window:Open")) -> (error out=w393:errorcluster)  [unwired: 1 in, 1 out]
                    n132 = call "Status Updated.vi"("Status"="Block Diagram shown." ("format string"), "Module ID"=w390) -> ()  [unwired: 9 in, 1 out]
                  }
                  frame True {
                    # "Password-protected VI, and the password is not in the cache. Do not show the diagram."
                  }
                }
              }
              frame condition #1 {
              }
            }
          }
          frame "--- Module Specific ---" {
            # "Separator -- The following cases handle messages specific to this Module."
            n133 = Merge Errors(w399) -> (w397:errorcluster)
          }
          frame "getISA010State" {
            n134 = Variant To Data(error in=w419, type=T6 {"Module ID"=-1, "Boolean"=FALSE, "state"=""} ("getISA010State Argument"), Variant=w418) -> (data=w416:T6, error out=w408:errorcluster)
            n135 = Unbundle By Name(w405) -> ("Serial Module ID"=w414:i32, "ISA010"=w410:refnum<class "ISA010.lvclass">, "ISACommands"=w403:string[], "ModBUS"=w400:refnum<class "ASCII.lvclass">)
            n136 = Unbundle By Name(w416) -> ()  [unwired: 2 out]
            n137 = call-dynamic "collectFrame.vi"("Reset"=TRUE, "error in (no error)"=w408, "byte"=u8 0, "ASCII in"=w400) -> ("error out"=w409:errorcluster)  [unwired: 3 in, 4 out]
            n138 = call "getState.vi"("error in (no error)"=w409, "ISA010 in"=w410) -> ("error out"=w411:errorcluster, "ISA010State"=w413:string)  [unwired: 7 in, 1 out]
            n139 = Build Array (concatenate)(w403, "getState" ("ISACommand")) -> (w402:string[])
            n140 = String To Byte Array(string=w413) -> (unsigned byte array=w412:u8[])
            n141 = call "Send.vi"("error in (no error)"=w411, "Bytes"=w412, "Module ID"=w414) -> ("error out"=w415:errorcluster)  [unwired: 8 in]
            n142 = Bundle By Name(cluster=w405, "ISACommands"=w402) -> (w404:T4)
          }
          frame "getOutputsForBitSet" {
            n143 = Unbundle By Name(w432) -> ("Serial Module ID"=w436:i32, "ISACommands"=w430:string[], "ModBUS"=w427:refnum<class "ASCII.lvclass">)  [unwired: 1 out]
            n144 = call-dynamic "collectFrame.vi"("Reset"=TRUE, "error in (no error)"=w438, "byte"=u8 0, "ASCII in"=w427) -> ("error out"=w425:errorcluster, "ASCII out"=w426:refnum<class "ASCII.lvclass">)  [unwired: 3 in, 3 out]
            n145 = call-dynamic "0x03ReadHoldingRegisters.vi"("Length 2"=u16 1, "error in (no error)"=w425, "Register"=u16 2, "Addressc"=u8 1, "ASCII in"=w426) -> ("error out"=w424:errorcluster, "Frame"=w423:string)  [unwired: 4 in, 1 out]
            n146 = Build Array (concatenate)(w430, "getOutputsForBitSet" ("ISACommand")) -> (w429:string[])
            n147 = String To Byte Array(string=w423) -> (unsigned byte array=w435:u8[])
            n148 = call "Send.vi"("error in (no error)"=w424, "Bytes"=w435, "Module ID"=w436) -> ("error out"=w437:errorcluster)  [unwired: 8 in]
            n149 = Bundle By Name(cluster=w432, "ISACommands"=w429) -> (w431:T4)
          }
          frame "setPWM" {
            n150 = Unbundle By Name(w453) -> ("ISACommands"=w449:string[], "ModBUS"=w454:refnum<class "ASCII.lvclass">, "Serial Module ID"=w440:i32)  [unwired: 1 out]
            n151 = Variant To Data(error in=w461, type=T7 {"Module ID"=-1, "PWM"=0} ("setPWM Argument"), Variant=w460) -> (data=w458:T7, error out=w455:errorcluster)
            n152 = Unbundle By Name(w458) -> ("PWM"=w443:u8)  [unwired: 1 out]
            n153 = call-dynamic "collectFrame.vi"("Reset"=TRUE, "error in (no error)"=w455, "byte"=u8 0, "ASCII in"=w454) -> ("error out"=w444:errorcluster, "ASCII out"=w445:refnum<class "ASCII.lvclass">)  [unwired: 3 in, 3 out]
            n154 = Build Array (concatenate)(w449, "setPWM" ("ISACommand")) -> (w450:string[])
            n155 = call-dynamic "0x06PresetSingleRegister.vi"("Data"=w443, "error in (no error)"=w444, "Register"=u16 5, "Addressc"=u8 1, "ASCII in"=w445) -> ("error out"=w441:errorcluster, "Frame"=w442:string)  [unwired: 4 in, 1 out]
            n156 = Bundle By Name(cluster=w453, "ISACommands"=w450) -> (w452:T4)
            n157 = String To Byte Array(string=w442) -> (unsigned byte array=w448:u8[])
            n158 = call "Send.vi"("error in (no error)"=w441, "Bytes"=w448, "Module ID"=w440) -> ("error out"=w439:errorcluster)  [unwired: 8 in]
          }
          frame "OutputCommand" {
            n159 = Unbundle By Name(w478) -> ("ISACommands"=w474:string[], "ModBUS"=w479:refnum<class "ASCII.lvclass">, "outputCommand"=w464:string, "Serial Module ID"=w466:i32, "outputs"=w463:u16)
            n160 = call-dynamic "collectFrame.vi"("Reset"=TRUE, "error in (no error)"=w482, "byte"=u8 0, "ASCII in"=w479) -> ("error out"=w469:errorcluster, "ASCII out"=w470:refnum<class "ASCII.lvclass">)  [unwired: 3 in, 3 out]
            n161 = case shown="\"setKASAWAR_H\"" w464 {
              tunnel: w463 -> [w483 w486 w490 w493 w497]
              tunnel: [w483 w484 w488 w491 w495] -> w462
              frame Default {
              }
              frame "setDKG_H" {
                n162 = Or(x=w486, y=u16 1) -> (x .or. y?=w484:u16)
              }
              frame "setDKG_L" {
                n163 = Not(x=u16 1 ("y")) -> (.not. x?=w487:u16)
                n164 = And(x=w490, y=w487) -> (x .and. y?=w488:u16)
              }
              frame "setKASAWAR_H" {
                n165 = Or(x=w493, y=u16 2) -> (x .or. y?=w491:u16)
              }
              frame "setKASAWAR_L" {
                n166 = Not(x=u16 2 ("y")) -> (.not. x?=w494:u16)
                n167 = And(x=w497, y=w494) -> (x .and. y?=w495:u16)
              }
            }
            n168 = Build Array (concatenate)(w474, "OutputCommand" ("ISACommand")) -> (w475:string[])
            n169 = call-dynamic "0x06PresetSingleRegister.vi"("Data"=w462, "error in (no error)"=w469, "Register"=u16 2, "Addressc"=u8 1, "ASCII in"=w470) -> ("error out"=w467:errorcluster, "Frame"=w468:string)  [unwired: 4 in, 1 out]
            n170 = Bundle By Name(cluster=w478, "ISACommands"=w475) -> (w477:T4)
            n171 = String To Byte Array(string=w468) -> (unsigned byte array=w473:u8[])
            n172 = call "Send.vi"("error in (no error)"=w467, "Bytes"=w473, "Module ID"=w466) -> ("error out"=w465:errorcluster)  [unwired: 8 in]
          }
          frame "SetServiceMode" {
            n173 = Unbundle By Name(w516) -> ("ISACommands"=w512:string[], "ModBUS"=w517:refnum<class "ASCII.lvclass">, "Serial Module ID"=w504:i32)  [unwired: 1 out]
            n174 = Variant To Data(error in=w523, type=T8 {"Module ID"=-1, "SET"=FALSE} ("SetServiceMode Argument"), Variant=w522) -> (data=w521:T8, error out=w518:errorcluster)
            n175 = Unbundle By Name(w521) -> ("SET"=w501:bool)  [unwired: 1 out]
            n176 = call-dynamic "collectFrame.vi"("Reset"=TRUE, "error in (no error)"=w518, "byte"=u8 0, "ASCII in"=w517) -> ("error out"=w507:errorcluster, "ASCII out"=w508:refnum<class "ASCII.lvclass">)  [unwired: 3 in, 3 out]
            n177 = Select(t=u16 7493, s=w501, f=u16 1111) -> (s? t:f=w498:u16)
            n178 = Build Array (concatenate)(w512, "setServiceMode" ("ISACommand")) -> (w513:string[])
            n179 = call-dynamic "0x06PresetSingleRegister.vi"("Data"=w498, "error in (no error)"=w507, "Register"=u16 1, "Addressc"=u8 1, "ASCII in"=w508) -> ("error out"=w505:errorcluster, "Frame"=w506:string)  [unwired: 4 in, 1 out]
            n180 = Bundle By Name(cluster=w516, "ISACommands"=w513) -> (w515:T4)
            n181 = String To Byte Array(string=w506) -> (unsigned byte array=w511:u8[])
            n182 = call "Send.vi"("error in (no error)"=w505, "Bytes"=w511, "Module ID"=w504) -> ("error out"=w503:errorcluster)  [unwired: 8 in]
          }
          frame "setDKG" {
            n183 = Variant To Data(error in=w538, type=T9 {"Module ID"=-1, "DKG"=FALSE} ("setDKG Argument"), Variant=w536) -> (data=w534:T9, error out=w528:errorcluster)
            n184 = Unbundle By Name(w534) -> ("DKG"=w532:bool)
            n185 = Select(t="setDKG_H" ("outputCommand"), s=w532, f="setDKG_L" ("outputCommand")) -> (s? t:f=w529:string)
            n186 = Bundle By Name(cluster=w537, "outputCommand"=w529) -> (w533:T4)
            n187 = call-poly <vilib>:"Delacor_lib_QMH_Enqueue Message (poly).vi"("Priority Message? (F)"=TRUE, "error in (no error)"=w528, "Message"="getOutputsForBitSet" ("outputCommand"), "Message Queue in"=w525) -> ("error out"=w527:errorcluster)  [unwired: 6 in, 1 out]
          }
          frame "setKASAWAR" {
            n188 = Variant To Data(error in=w553, type=T10 {"Module ID"=-1, "KASAWAR"=FALSE} ("setKASAWAR Argument"), Variant=w551) -> (data=w550:T10, error out=w546:errorcluster)
            n189 = Unbundle By Name(w550) -> ("KASAWAR"=w548:bool)
            n190 = Select(t="setKASAWAR_H" ("outputCommand"), s=w548, f="setKASAWAR_L" ("outputCommand")) -> (s? t:f=w547:string)
            n191 = Bundle By Name(cluster=w552, "outputCommand"=w547) -> (w549:T4)
            n192 = call-poly <vilib>:"Delacor_lib_QMH_Enqueue Message (poly).vi"("Priority Message? (F)"=TRUE, "error in (no error)"=w546, "Message"="getOutputsForBitSet" ("outputCommand"), "Message Queue in"=w543) -> ("error out"=w545:errorcluster)  [unwired: 6 in, 1 out]
          }
          frame "Config" {
            w558 = ""
            n193 = Unbundle By Name(w570) -> ("Serial Module ID"=w569:i32)
            n194 = Variant To Data(error in=w574, type=T11 {"Module ID"=-1, "ConfigJson"=""} ("Config Argument"), Variant=w573) -> (data=w571:T11, error out=w567:errorcluster)
            n195 = Unbundle By Name(w571) -> ("ConfigJson"=w556:string)
            n196 = Unflatten From JSON(path=string[] ["MQTT"], JSON string=w556, type and defaults=w558) -> (value=w554:string, error out=w559:errorcluster)  [unwired: 4 in]
            n197 = Unflatten From JSON(path=string[] ["MOXA"], JSON string=w556, type and defaults=w558, error in (no error)=w559) -> (value=w555:string)  [unwired: 3 in, 1 out]
            n198 = call "config.vi"("error in (no error)"=w567, "config"=w555, "Module ID"=w569) -> ("error out"=w568:errorcluster)  [unwired: 8 in]
            n199 = call "Open.vi"("error in (no error)"=w568, "Module ID"=w569) -> ("error out"=w563:errorcluster)  [unwired: 9 in]
            n200 = call-poly <vilib>:"Delacor_lib_QMH_Enqueue Message (poly).vi"("error in (no error)"=w563, "Message"="SetServiceMode", "Message Queue in"=w562) -> ("error out"=w561:errorcluster)  [unwired: 7 in, 1 out]
            n201 = call "configMQTT.vi"("error in (no error)"=w561, "conf(empty for default)"=w554, "Module ID"=w565) -> ("error out"=w566:errorcluster)  [unwired: 8 in]
          }
          frame "---Copy This Frame---" {
            # "Duplicate this frame when creating new messages.  Change this comment in the duplicated frame to describe this message."
            n202 = Merge Errors(w577) -> (w575:errorcluster)
          }
          frame "ModbusReply" {
            # "Duplicate this frame when creating new messages.  Change this comment in the duplicated frame to describe this message."
            n203 = Unbundle By Name(w590) -> ("ISACommands"=w592:string[], "ISA010"=w582:refnum<class "ISA010.lvclass">)
            n204 = property class="Mod Admin"(reference=w585) -> ("Accessors:Module ID"=w584:i32)  [unwired: 1 in, 2 out]
            n205 = Delete From Array(array=w592, length=1) -> (deleted portion=w588:string[], array with subset deleted=w589:string[])  [unwired: 1 in]
            n206 = Index Array(array=w588) -> (element=w587:string)  [unwired: 1 in]
            n207 = Bundle By Name(cluster=w590, "ISACommands"=w589) -> (w579:T4)
            n208 = case shown="\"getState\"" w587 {
              selector: w587 -> [w595 _ _]
              tunnel: w586 -> [w598 w608 w620]
              tunnel: w584 -> [w596 _ w621]
              tunnel: w583 -> [_ w609 w618]
              tunnel: w582 -> [_ _ w615]
              tunnel: [w597 w602 w611] -> w581
              tunnel: [w594 w605 w613] -> w580
              tunnel: w579 -> [w594 w606 w613]
              tunnel: w578 -> [_ w600 _]
              frame Default {
                n209 = call "ISA010State.vi"("error in (no error)"=w598, "state"=w595, "Module ID"=w596) -> ("error out"=w597:errorcluster)  [unwired: 8 in]
              }
              frame "getOutputsForBitSet" {
                n210 = Variant To Data(error in=w608, type=i16[] [] ("Data"), Variant=w609) -> (data=w607:i16[], error out=w603:errorcluster)
                n211 = Index Array(array=w607) -> (element=w604:i16)  [unwired: 1 in]
                n212 = Bundle By Name(cluster=w606, "outputs"=w604) -> (w605:T4)
                n213 = call-poly <vilib>:"Delacor_lib_QMH_Enqueue Message (poly).vi"("Priority Message? (F)"=TRUE, "error in (no error)"=w603, "Message"="OutputCommand", "Message Queue in"=w600) -> ("error out"=w602:errorcluster)  [unwired: 6 in, 1 out]
              }
              frame "getState" {
                n214 = Variant To Data(error in=w620, type=i16[] [] ("Data"), Variant=w618) -> (data=w616:i16[], error out=w617:errorcluster)
                n215 = call-dynamic "decodeState.vi"("error in (no error)"=w617, "Data"=w616, "ISA010 in"=w615) -> ("error out"=w614:errorcluster, "JSON string"=w612:string)  [unwired: 6 in, 1 out]
                n216 = call "ISA010State.vi"("error in (no error)"=w614, "state"=w612, "Module ID"=w621) -> ("error out"=w611:errorcluster)  [unwired: 8 in]
              }
            }
            n217 = Merge Errors(w581, w586) -> (w593:errorcluster)
          }
          frame "--- Exit and Error Handling---" {
            # "Separator - the following cases handle errors and exit messages."
            n218 = Merge Errors(w624) -> (w622:errorcluster)
          }
          frame "Error" {
            # "#CodeRecommended - If you ever change the name of this \"Error\" message, you'll need to update the name in the Check Loop Error.vi as well."
            # "#CodeRecommended - If the module is running in standalone mode (External Launch = FALSE), this code will pop up an error dialog and call the 'Exit' message if an error occurs. Add more fine-grained error handling here."
            # "Error - Check the error message data and respond accordingly. This message is sent by the \"Error Handler\" VIs at the end of each loop in this application."
            n219 = property class="Mod Admin"(reference=w630) -> ("Accessors:External Launch"=w627:bool, "Accessors:Module ID"=w629:i32)  [unwired: 1 in, 2 out]
            n220 = Variant To Data(error in=w635, type=errorcluster {"status"=FALSE, "code"=0, "source"=""} ("error constant"), Variant=w633) -> (data=w636:errorcluster, error out=w631:errorcluster)
            n221 = call "Error Reported.vi"("Error"=w636, "Module ID"=w629) -> ()  [unwired: 9 in, 1 out]
            n222 = case shown="False" w627 {
              tunnel: [w641 _] -> w628
              tunnel: w626 -> [w640 _]
              tunnel: w636 -> [w637 _]
              frame False {
                # "If the module is running standalone, then pop up an error dialog and call the \"Exit\" message."
                n223 = call <vilib>:"Simple Error Handler.vi"("error in (no error)"=w637) -> ()  [unwired: 4 in, 5 out]
                n224 = call-poly <vilib>:"Delacor_lib_QMH_Enqueue Message (poly).vi"("Priority Message? (F)"=TRUE, "Message"="Exit", "Message Queue in"=w640) -> ("error out"=w641:errorcluster)  [unwired: 7 in, 1 out]
              }
              frame True {
                # "If the module was launched externally, calling the Error Reported broadcast VI is the only action performed by the \"Error\" message. The module's caller can then process the error appropriately."
              }
            }
            n225 = Merge Errors(w631, w628) -> (w625:errorcluster)
            n226 = local write "error out"(w625) -> ()
          }
          frame "Simulate MHL Error" {
            # "Simulate an error occurring at the MHL"
            n227 = property class="Mod Admin"(reference=w643) -> ("Accessors:Module ID"=w644:i32)  [unwired: 1 in, 2 out]
            n228 = call "Module Name--constant.vi"("Module ID"=w644) -> ("Module Name"=w642:string)  [unwired: 10 in]
            n229 = xnode "Error Ring"("parameter 0"=w642) -> ("error out"=w645:errorcluster)
            n230 = Merge Errors(w648, w645) -> (w646:errorcluster)
          }
          frame "Confirm Quit" {
            # "#CodeNeeded - If you want to provide an \"Are you sure\" dialog (or some other notification) before the application exits, place that code here. This message is typically sent from a Panel Close? event."
            # "Confirm Quit - Message that can confirm whether or not the user wants to exit this instance."
            n231 = call-poly <vilib>:"Delacor_lib_QMH_Enqueue Message (poly).vi"("Priority Message? (F)"=TRUE, "error in (no error)"=w658, "Message"="Exit", "Message Queue in"=w659) -> ("error out"=w661:errorcluster)  [unwired: 6 in, 1 out]
            n232 = Merge Errors(w661) -> (w657:errorcluster)
          }
          frame "Exit" {
            w677 = 91  # 91: not all Exit messages will have an argument
            w680 = TRUE  # Stop the VI
            # "Release the message queue reference"
            # "#CodeNeeded - Add any required cleanup code here"
            # "Exit - Exit the application."
            n233 = Variant To Data(error in=w683, type=T5 {"Origin"="", "Module ID"=-1, "Exit via Stop Module Req?"=FALSE, "Wait for Module to stop?"=FALSE} ("Stop Argument"), Variant=w675) -> (data=w672:T5, error out=w676:errorcluster)
            n234 = Unbundle By Name(w668) -> ("Serial Module ID"=w666:i32)
            n235 = call <vilib>:"Clear Errors.vi"("error in (no error)"=w676, "specific error code to clear (0: all)"=w677) -> ("error out"=w682:errorcluster)  [unwired: 4 in, 1 out]
            n236 = control-ref of="This VI"() -> (w670:refnum<vi>)
            n237 = call-dynamic "Delacor_lib_QMH_Release Message Queue.vi"("error in (no error)"=w682, "Message Queue"=w681) -> ("error out"=w669:errorcluster)  [unwired: 9 in]
            n238 = call "Handle Exit.vi"("Stop Argument"=w672, "Module Admin in"=w671, "VI reference"=w670) -> ("error out"=w678:errorcluster, "Wait for Stop?"=w673:bool)  [unwired: 7 in]
            n239 = call "close.vi"("error in (no error)"=w669, "Module ID"=w666) -> ("error out"=w667:errorcluster)  [unwired: 9 in]
            n240 = call "Stop Module.vi"("error in (no error)"=w667, "Module ID"=w666) -> ("error out"=w663:errorcluster)  [unwired: 9 in]
            n241 = disable-structure shown="Enabled" {
              disable-tunnel: [w687 w688] -> w665
              disable-tunnel: w664 -> [w685 _]
              disable-tunnel: w663 -> [w684 w688]
              frame Enabled {
                n242 = call "disconnect.vi"("error in (no error)"=w684, "Module ID"=w685) -> ("error out"=w686:errorcluster)  [unwired: 9 in]
                n243 = call "Stop Module.vi"("error in (no error)"=w686, "Module ID"=w685) -> ("error out"=w687:errorcluster)  [unwired: 9 in]
              }
              frame Disabled {
              }
            }
            n244 = Merge Errors(w678, w665) -> (w679:errorcluster)
          }
          frame Default {
            # "'Default' case only runs if there is a message that isn't defined in any of the other cases.  Output a programming error."
            n245 = property class="Mod Admin"(reference=w690) -> ("Accessors:Module ID"=w689:i32)  [unwired: 1 in, 2 out]
            n246 = call "Module Name--constant.vi"("Module ID"=w689) -> ("Module Name"=w691:string)  [unwired: 10 in]
            n247 = xnode "Error Ring"("parameter 0"=w692, "parameter 1"=w691) -> ("error out"=w693:errorcluster)
          }
        }
        n248 = call-dynamic "Delacor_lib_QMH_Error Handler - Message Handling Loop.vi"("error in (no error)"=w329, "Message Queue in"=w320) -> ("dup error in"=w319:errorcluster)  [unwired: 8 in, 1 out]
      }
    }
    frame Error {
      n249 = call "Synchronize Caller Events.vi"("Module Admin"=w705) -> ("Module Admin out"=w704:refnum<class "Delacor_lib_QMH_Cloneable Module Admin.lvclass">)  [unwired: 9 in, 1 out]
      n250 = property class="Mod Admin"(reference=w704) -> ("Accessors:Module ID"=w703:i32)  [unwired: 1 in, 2 out]
      n251 = call "Module Name--constant.vi"("Module ID"=w703) -> ("Module Name"=w708:string)  [unwired: 10 in]
      n252 = call "Remove.vi"("Module ID"=w703) -> ()  [unwired: 9 in, 2 out]
      n253 = Format Into String(format string="An error occurred during initialization. %s is no longer running.", w708) -> (resulting string=w706:string)  [unwired: 2 in, 1 out]
      n254 = call "Error Reported.vi"("Additional Information"=w706, "Error"=w709, "Module ID"=w703) -> ()  [unwired: 8 in, 1 out]
    }
  }
  n255 = Merge Errors(w28, w27) -> (w29:errorcluster)
  n256 = call "Close Module.vi"("error in (no error)"=w29, "Wait for stop?"=w19, "Module Admin in"=w21) -> ("error out"=w23:errorcluster, "External Launch"=w17:bool, "Module Admin out"=w20:refnum<class "Delacor_lib_QMH_Cloneable Module Admin.lvclass">)  [unwired: 6 in]
  n257 = Unregister For Events(event registration refnum=w26, error in=w23) -> (error out=w18:errorcluster)
  "error out" <- w18
  n258 = local write "Module Admin"(w20) -> ()
  n259 = case "External Launch?" shown="True" w17 {
    tunnel: w18 -> [_ w711]
    frame False {
    }
    frame True {
      n260 = case shown="No Error" w711 {
        frame No Error {
          n261 = invoke class="VI" method="FP.Close"() -> ()  [unwired: 3 in, 3 out]
        }
        frame Error {
          n262 = invoke class="VI" method="FP.Open"("Activate"=TRUE ("Activate?")) -> ()  [unwired: 4 in, 5 out]
        }
      }
    }
  }
